vi "balloon入队列.vi"(7 "队列":refnum<queue>, 8 "故障详情":string, 9 "告警信息":string, 10 "故障信息":string, 11 "参数名称":string) -> (3 "队列输出":refnum<queue>)   [LabVIEW 2016, in "环境动力监测库.lvlib" / "AIRMAR WeatherCaster.lvlib"]
uses:
  AIRMAR WeatherCaster.lvlib
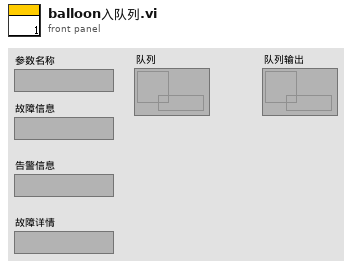
[diagram p1: front panel]
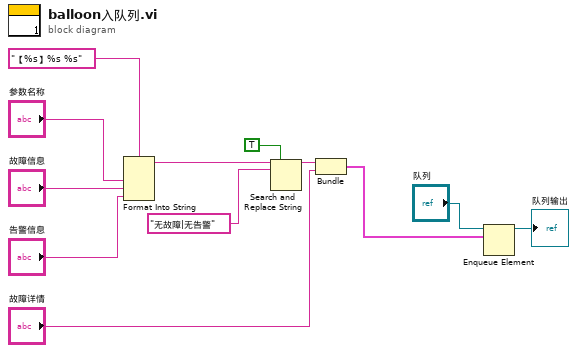
[diagram p0: block diagram]
diagram:
  n1 = Format Into String(format string="【%s】%s %s" ("格式字符串"), "参数名称", "故障信息", "告警信息") -> (resulting string=w11:string)  [unwired: 2 in, 1 out]
  n2 = Search and Replace String(replace all?=TRUE ("替换全部？(F)"), input string=w11, search string="无故障|无告警" ("字符串")) -> (result string=w12:string)  [unwired: 5 in, 3 out]
  n3 = Bundle("result string"=w12, "故障详情"="故障详情") -> (w3:cluster{"result string":string, "故障详情":string})  [unwired: 1 in]
  n4 = Enqueue Element(queue="队列", element=w3) -> (queue out=→"队列输出":refnum<queue>)  [unwired: 2 in, 2 out]
